vi "OAT Set Orbit Plot Property.vi"(6 "max value":dbl format="%.2f", 7 "orbit plot ref":refnum<vi>, 8 "error in (no error)":errorcluster, 10 "reset? (F)":bool, 11 "XY plot data in":cluster{dbl[], dbl[]}[](array[cluster]) {"?" format="%.2f"; "?" format="%.2f"}) -> (0 "error out":errorcluster, 3 "XY plot data out":cluster{dbl[], dbl[]}[](array[cluster]) {"?" format="%.2f"; "?" format="%.2f"}, 5 "orbit plot ref":refnum<vi>)   [LabVIEW 2017]
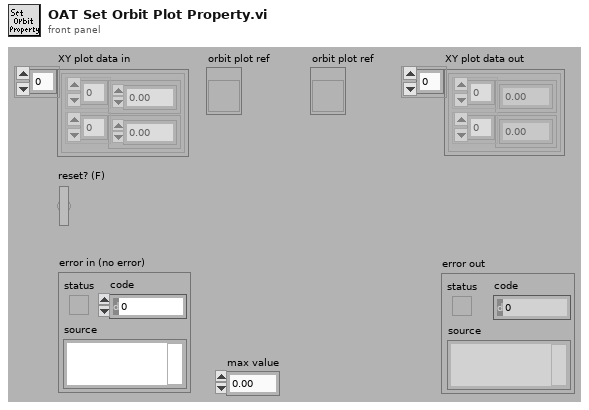
[diagram p1: front panel]
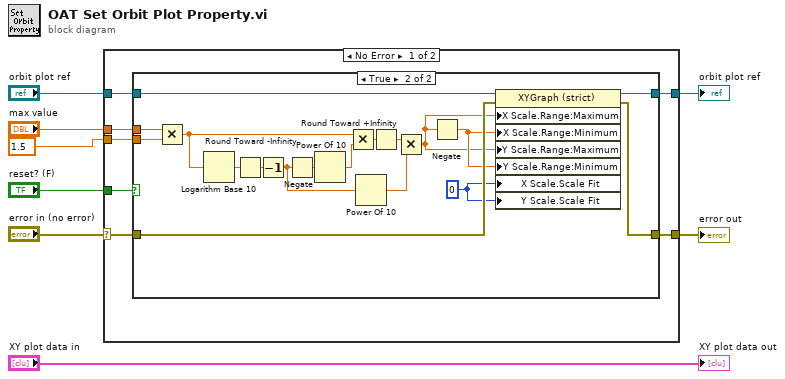
[diagram p0: block diagram]
diagram:
  n1 = case shown="No Error" "error in (no error)" {
    selector: "error in (no error)" -> [w11 w36]
    tunnel: "orbit plot ref" -> [w15 w37]
    tunnel: "max value" -> [w14 _]
    tunnel: 1.5 ("y") -> [w13 _]
    tunnel: [w12 w37] -> w4
    tunnel: [w10 w36] -> w2
    tunnel: "reset? (F)" -> [w9 _]
    frame No Error {
      n2 = case shown="True" w9 {
        tunnel: w15 -> [w16 w35]
        tunnel: w14 -> [_ w34]
        tunnel: w13 -> [_ w33]
        tunnel: [w16 w32] -> w12
        tunnel: w11 -> [w17 w31]
        tunnel: [w17 w30] -> w10
        frame False {
        }
        frame True {
          w28 = u8 0 ("X Scale.Scale Fit")
          n3 = Multiply(x=w34, y=w33) -> (x*y=w25:dbl)
          n4 = Logarithm Base 10(1:w25) -> (0:w22:dbl)
          n5 = Round Toward -Infinity(1:w22) -> (0:w20:dbl)
          n6 = Decrement(x=w20) -> (x-1=w19:dbl)
          n7 = Negate(x=w19) -> (-x=w27:dbl)
          n8 = Power Of 10(x=w27) -> (10^x=w26:dbl)
          n9 = Multiply(x=w25, y=w26) -> (x*y=w23:dbl)
          n10 = Power Of 10(x=w19) -> (10^x=w21:dbl)
          n11 = Round Toward +Infinity(x=w23) -> (ceil(x): smallest int >= x=w24:dbl)
          n12 = Multiply(x=w24, y=w21) -> (x*y=w18:dbl)
          n13 = Negate(x=w18) -> (-x=w29:dbl)
          n14 = property class="XYGraph (strict)"(reference=w35, error in=w31, "X Scale.Range:Maximum"=w18, "X Scale.Range:Minimum"=w29, "Y Scale.Range:Maximum"=w18, "Y Scale.Range:Minimum"=w29, "X Scale.Scale Fit"=w28, "Y Scale.Scale Fit"=w28) -> (reference out=w32:refnum<vi>, error out=w30:errorcluster)
        }
      }
    }
    frame Error {
    }
  }
  "orbit plot ref" <- w4
  "error out" <- w2
  "XY plot data out" <- "XY plot data in"
